vi "Read Execution time.vi"(11 "Method Result In":T1) -> (1 "Execution time string":string, 2 "Execution time":dbl, 3 "Method Result Out":T1)   [LabVIEW 2020, in "Method Result.lvlib"]
uses:
  Method Result.lvlib
  Method Result.ctl
  Rewrite Project/Result/Status.ctl
  Assertion Result/Assertion Result.ctl
  Assertion Result/Public/TypeDefs/Assertion Type.ctl
  Assertion Result/Assertion Result.lvlib
  Rewrite Project/Result/Result.lvlib
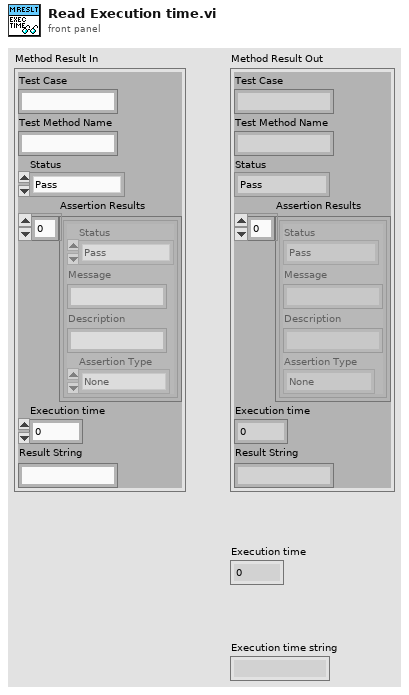
[diagram p1: front panel]
types:
  T1 = typedef "Method Result.lvlib/Method Result.ctl" = cluster{"Test Case":string, "Test Method Name":string, "Status":T2, "Assertion Results":T3[], "Execution time":dbl, "Result String":string}
  T2 = typedef "Result.lvlib/Status.ctl" = enum16{"Pass", "Fail", "Error", "Skipped", "Setup Error", "Broken", "Teardown Error"}
  T3 = typedef "Assertion Result.lvlib/Assertion Result.ctl" = cluster{"Status":T2, "Message":string, "Description":string, "Assertion Type":T4}
  T4 = typedef "Result.lvlib/Assertion Type.ctl" = enum16{"None", "Pass", "Fail", "Skip", "Pass if Equal", "Fail if Equal", "Pass if Error", "Fail if Error", "Pass if", "Fail if"}
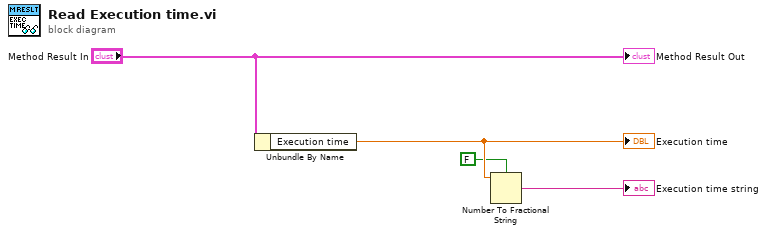
[diagram p0: block diagram]
diagram:
  n1 = Unbundle By Name("Method Result In") -> ("Execution time"=w3:dbl)
  "Execution time" <- w3
  n2 = Number To Fractional String(use system decimal point (T)=FALSE, number=w3) -> (F-format string=→"Execution time string":string)  [unwired: 2 in]
  "Method Result Out" <- "Method Result In"
